vi "QPD_channels.vi"(8 "error in":errorcluster) -> (0 "error out":errorcluster, 3 "task out":refnum<k21>)   [LabVIEW 2019]
uses:
  global_VIs/Global_2.vi
  <vilib>/DAQmx/create/channels.llb/DAQmx Create Channel (AI-Voltage-Basic).vi
  <vilib>/DAQmx/configure/timing.llb/DAQmx Timing (Sample Clock).vi
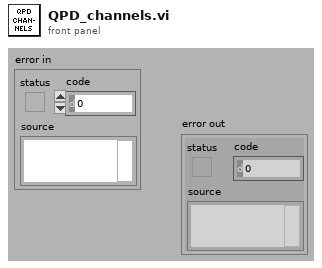
[diagram p1: front panel]
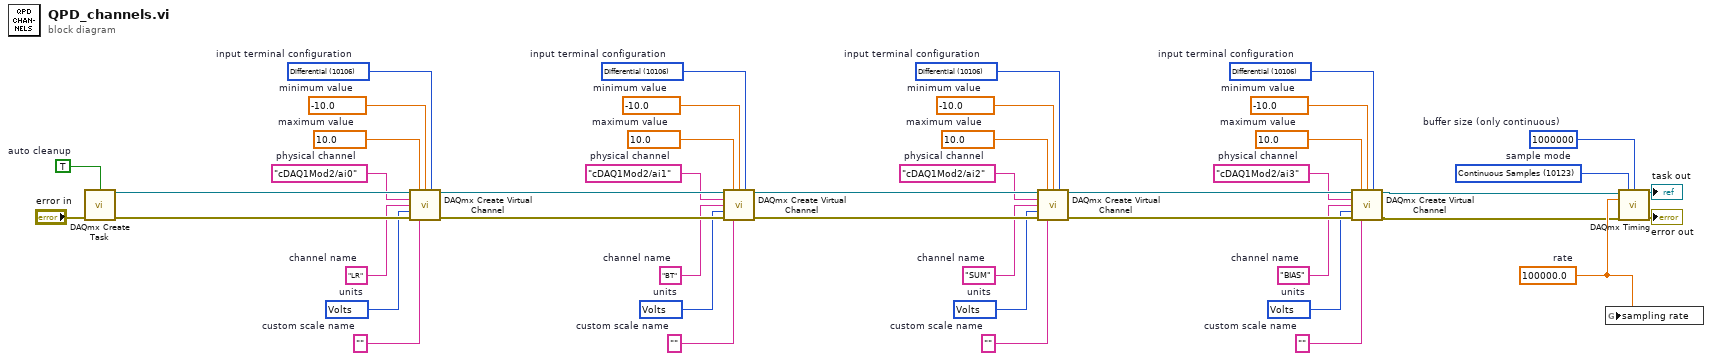
[diagram p0: block diagram]
diagram:
  w4 = 10123 items=["Finite Samples"=10178, "Continuous Samples"=10123, "Hardware Timed Single Point"=12522]  # sample mode
  w5 = 1000000  # buffer size (only continuous)
  w3 = 100000.0  # rate
  w8 = 10106 items=["default"=-1, "RSE"=10083, "NRSE"=10078, "Differential"=10106, "Pseudodifferential"=12529]  # input terminal configuration
  w9 = 10348 items=["Volts"=10348, "From Custom Scale"=10065]  # units
  w10 = "BIAS"  # channel name
  w11 = ""  # custom scale name
  w12 = -10.0  # minimum value
  w13 = 10.0  # maximum value
  w14 = "cDAQ1Mod2/ai3"  # physical channel
  w16 = 10106 items=["default"=-1, "RSE"=10083, "NRSE"=10078, "Differential"=10106, "Pseudodifferential"=12529]  # input terminal configuration
  w17 = 10348 items=["Volts"=10348, "From Custom Scale"=10065]  # units
  w18 = "SUM"  # channel name
  w20 = ""  # custom scale name
  w21 = -10.0  # minimum value
  w22 = 10.0  # maximum value
  w23 = "cDAQ1Mod2/ai2"  # physical channel
  w25 = 10106 items=["default"=-1, "RSE"=10083, "NRSE"=10078, "Differential"=10106, "Pseudodifferential"=12529]  # input terminal configuration
  w26 = 10348 items=["Volts"=10348, "From Custom Scale"=10065]  # units
  w27 = "BT"  # channel name
  w29 = ""  # custom scale name
  w30 = -10.0  # minimum value
  w31 = 10.0  # maximum value
  w32 = "cDAQ1Mod2/ai1"  # physical channel
  w34 = 10106 items=["default"=-1, "RSE"=10083, "NRSE"=10078, "Differential"=10106, "Pseudodifferential"=12529]  # input terminal configuration
  w35 = 10348 items=["Volts"=10348, "From Custom Scale"=10065]  # units
  w36 = "LR"  # channel name
  w38 = ""  # custom scale name
  w39 = -10.0  # minimum value
  w40 = 10.0  # maximum value
  w41 = "cDAQ1Mod2/ai0"  # physical channel
  w43 = TRUE  # auto cleanup
  n1 = call <vilib>:"DAQmx Create Task.vi"("auto cleanup"=w43, "error in"="error in") -> ("task out"=w42:refnum<k21>, "error out"=w44:errorcluster)  [unwired: 12 in]
  n2 = call-poly <vilib>:"DAQmx Create Virtual Channel.vi"("task in"=w42, "maximum value"=w40, "minimum value"=w39, "input terminal configuration"=w34, "physical channels"=w41, "name to assign"=w36, "units"=w35, "error in"=w44, "custom scale name"=w38) -> ("task out"=w33:refnum<k21>, "error out"=w37:errorcluster)  [unwired: 5 in]
  n3 = call-poly <vilib>:"DAQmx Create Virtual Channel.vi"("task in"=w33, "maximum value"=w31, "minimum value"=w30, "input terminal configuration"=w25, "physical channels"=w32, "name to assign"=w27, "units"=w26, "error in"=w37, "custom scale name"=w29) -> ("task out"=w24:refnum<k21>, "error out"=w28:errorcluster)  [unwired: 5 in]
  n4 = call-poly <vilib>:"DAQmx Create Virtual Channel.vi"("task in"=w24, "maximum value"=w22, "minimum value"=w21, "input terminal configuration"=w16, "physical channels"=w23, "name to assign"=w18, "units"=w17, "error in"=w28, "custom scale name"=w20) -> ("task out"=w15:refnum<k21>, "error out"=w19:errorcluster)  [unwired: 5 in]
  n5 = call-poly <vilib>:"DAQmx Create Virtual Channel.vi"("task in"=w15, "maximum value"=w13, "minimum value"=w12, "input terminal configuration"=w8, "physical channels"=w14, "name to assign"=w10, "units"=w9, "error in"=w19, "custom scale name"=w11) -> ("task out"=w2:refnum<k21>, "error out"=w1:errorcluster)  [unwired: 5 in]
  n6 = global write "Global_2.vi" "sampling rate"(w3) -> ()
  n7 = call-poly <vilib>:"DAQmx Timing.vi"("task/channels in"=w2, "sample mode"=w4, "samples per channel"=w5, "rate"=w3, "error in"=w1) -> ("task out"=→"task out":refnum<k21>, "error out"=→"error out":errorcluster)  [unwired: 9 in]
